vi "StandardStateMachine 1.vi"() -> ()   [LabVIEW 2012]
doc: "Use this template to build a standard state machine design pattern. Each state executes code and determines which state to transition to. Contrast this design pattern with the User Interface Event Handler pattern, in which code executes in response to user actions. Contrast this design pattern also with the Queued Message Handler pattern, in which each message handling code can queue zero or more new messages.\nNote: This template does not contain the most recent programming guidelines recommended by National Instruments. For a complete, project-based implementation of the Standard State Machine pattern, use the Create Project dialog box instead of this template."
uses:
  StateMachineStates 1.ctl
panel:
  out "Current State":i32
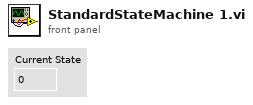
[diagram p1: front panel]
types:
  T1 = typedef "StateMachineStates 1.ctl" = enum16{"Initialize", "Stop", "State 1", "State 2"}
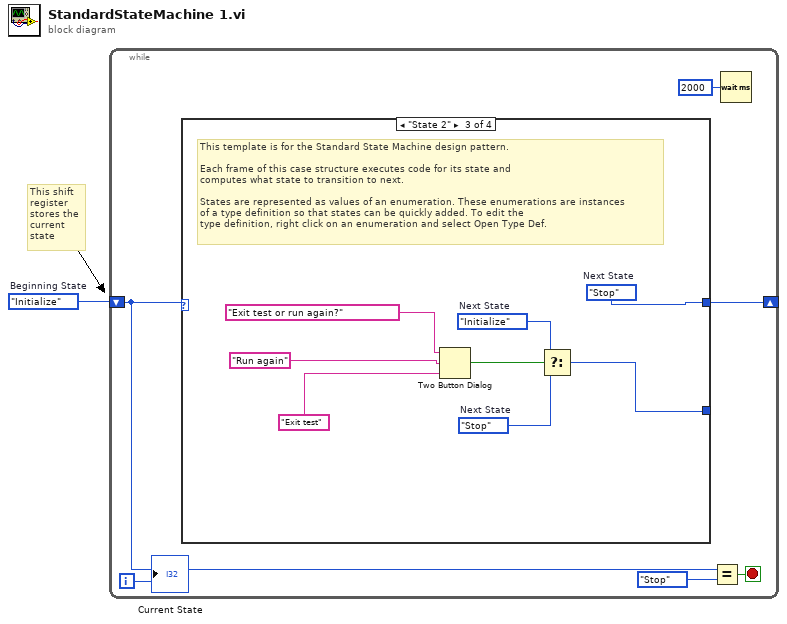
[diagram p0: block diagram]
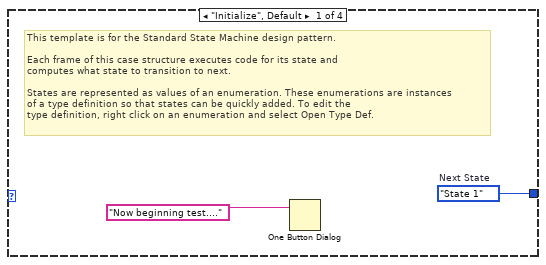
[diagram p2: hidden frame]
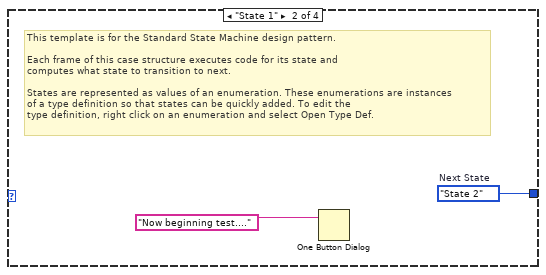
[diagram p3: hidden frame]
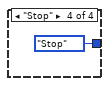
[diagram p4: hidden frame]
diagram:
  w1 = StateMachineStates_1."Initialize"  # Beginning State
  # "This shift\nregister\nstores the\ncurrent\nstate"
  n1 = while {
    shift-right: [w4] -> _
    shift-left: w1 -> [w5]
    i -> [w2]
    stop <- w7 stop-if-true
    n2 = case shown="\"State 2\"" w5 {
      tunnel: [w9 w11 w19 StateMachineStates_1."Stop" ("Next State")] -> w4
      tunnel: [_ _ w12 _] -> _
      frame "Initialize", Default {
        w9 = StateMachineStates_1."State 1"  # Next State
        # "This template is for the Standard State Machine design pattern.\n\nEach frame of this case structure executes code for its state and\ncomputes what state to transition to next.\n\nStates are represented as values of an enumeration. These enumerations are instances\nof a type definition so that states can be quickly added. To edit the \ntype definition, right click on an enumeration and select Open Type Def."
        n3 = One Button Dialog(message="Now beginning test....") -> ()  [unwired: 1 in, 1 out]
      }
      frame "State 1" {
        w11 = StateMachineStates_1."State 2"  # Next State
        # "This template is for the Standard State Machine design pattern.\n\nEach frame of this case structure executes code for its state and\ncomputes what state to transition to next.\n\nStates are represented as values of an enumeration. These enumerations are instances\nof a type definition so that states can be quickly added. To edit the \ntype definition, right click on an enumeration and select Open Type Def."
        n4 = One Button Dialog(message="Now beginning test....") -> ()  [unwired: 1 in, 1 out]
      }
      frame "State 2" {
        w18 = StateMachineStates_1."Initialize"  # Next State
        w17 = StateMachineStates_1."Stop"  # Next State
        w19 = StateMachineStates_1."Stop"  # Next State
        # "This template is for the Standard State Machine design pattern.\n\nEach frame of this case structure executes code for its state and\ncomputes what state to transition to next.\n\nStates are represented as values of an enumeration. These enumerations are instances\nof a type definition so that states can be quickly added. To edit the \ntype definition, right click on an enumeration and select Open Type Def."
        n5 = Two Button Dialog(message="Exit test or run again?", 1:"Exit test", 2:"Run again") -> (T button?=w16:bool)
        n6 = Select(t=w18, s=w16, f=w17) -> (s? t:f=w12:T1)
      }
      frame "Stop" {
      }
    }
    n7 = Equal?(x=w5, y=StateMachineStates_1."Stop" ("States")) -> (x = y?=w7:bool)
    n8 = Wait (ms)(milliseconds to wait=u32 2000) -> ()  [unwired: 1 out]
    "Current State" <- w2
  }
